vi "createILCCommunications.vi"(8 "error in (no error)":errorcluster, 11 "Boot in":refnum<class "Boot.lvclass">) -> (0 "error out":errorcluster, 2 "ILCCommunications":refnum<class "ILCCommunications.lvclass">, 3 "Boot out":refnum<class "Boot.lvclass">)   [LabVIEW 2016, in "Boot.lvclass"]
uses:
  Boot.lvclass
  ILCCommunications/ILCCommunications.lvclass
  ILCCommunications/ILCCommunications.lvclass/ILCCommunications.ctl
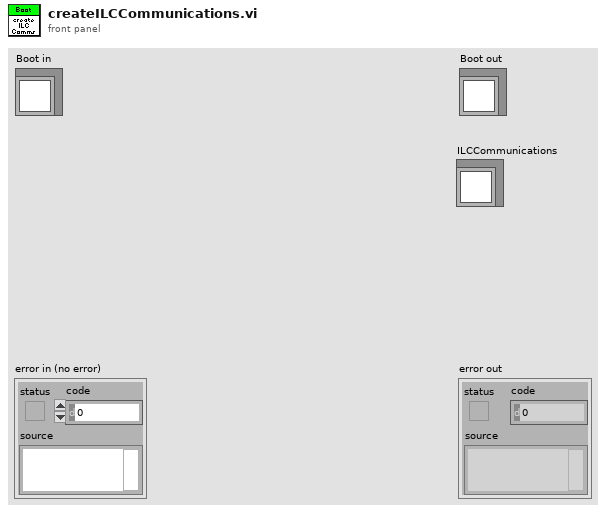
[diagram p1: front panel]
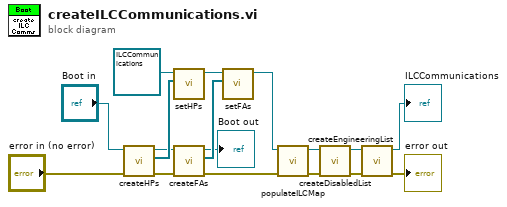
[diagram p0: block diagram]
diagram:
  n1 = call "createHPs.vi"("error in (no error)"="error in (no error)", "Boot in"="Boot in") -> ("error out"=w13:errorcluster, "HPs"=w17:refnum<class "HPILC.lvclass">[], "Boot out"=w12:refnum<class "Boot.lvclass">)  [unwired: 7 in]
  n2 = call "setHPs.vi"("HPs"=w17, "ILCCommunications in"=refnum<class "ILCCommunications.lvclass"> refnum ("ILCCommunications.lvclass")) -> ("ILCCommunications out"=w11:refnum<class "ILCCommunications.lvclass">)  [unwired: 9 in]
  n3 = call "createFAs.vi"("error in (no error)"=w13, "Boot in"=w12) -> ("error out"=w7:errorcluster, "FAs"=w10:refnum<class "FAILC.lvclass">[], "Boot out"=→"Boot out":refnum<class "Boot.lvclass">)  [unwired: 7 in]
  n4 = call "setFAs.vi"("FAs"=w10, "ILCCommunications in"=w11) -> ("ILCCommunications out"=w8:refnum<class "ILCCommunications.lvclass">)  [unwired: 9 in]
  n5 = call "populateILCMap.vi"("error in (no error)"=w7, "ILCCommunications in"=w8) -> ("error out"=w5:errorcluster, "ILCCommunications out"=w6:refnum<class "ILCCommunications.lvclass">)  [unwired: 8 in]
  n6 = call "createDisabledList.vi"("error in (no error)"=w5, "ILCCommunications in"=w6) -> ("error out"=w2:errorcluster, "ILCCommunications out"=w4:refnum<class "ILCCommunications.lvclass">)  [unwired: 8 in]
  n7 = call "createEngineeringList.vi"("error in (no error)"=w2, "ILCCommunications in"=w4) -> ("error out"=→"error out":errorcluster, "ILCCommunications out"=→"ILCCommunications":refnum<class "ILCCommunications.lvclass">)  [unwired: 8 in]
